vi "ProcessData.vi"() -> ()   [LabVIEW 2022 SP3]
panel:
  in  "Data Directory":path=path "C:/Users/LAV-UFSC-2023/Documents/LAV-TCC/Dados-Experimentos/Dados-Bancada-LABVIEW"
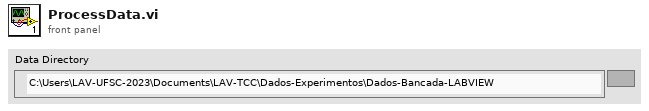
[diagram p1: front panel]
types:
  T1 = enum16{"open", "open or create", "create or replace", "create", "open (read-only)"}
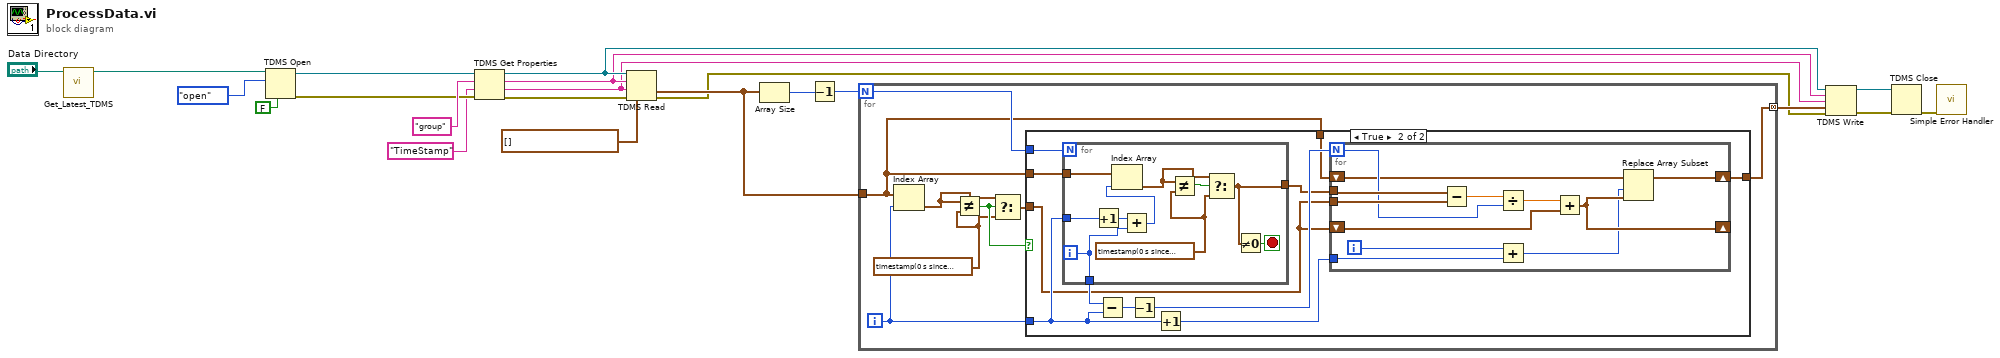
[diagram p0: block diagram]
diagram:
  n1 = call "Get_Latest_TDMS.vi"("Data Directory"="Data Directory") -> ("Latest_TDMS_File_Path"=w20:path)  [unwired: 10 in]
  n2 = TDMS Open(6:FALSE ("disable buffering? (T)"), 10:T1."open" ("operation (0:open)"), 11:w20) -> (0:w18:errorcluster, 3:w17:refnum<k34>)  [unwired: 4 in]
  n3 = TDMS Get Properties(8:w18, 9:"TimeStamp" ("group name (Untitled)"), 10:"group" ("group name (Untitled)"), 11:w17) -> (0:w13:errorcluster, 1:w5:string, 2:w7:string, 3:w8:refnum<k34>)  [unwired: 2 in, 2 out]
  n4 = TDMS Read(0:w8, 5:w7, 7:w5, 11:w13, 12:timestamp[] []) -> (10:w9:timestamp[], 15:w4:errorcluster)  [unwired: 3 in, 4 out]
  n5 = Array Size(array=w9) -> (size(s)=w11:i32)
  n6 = Decrement(x=w11) -> (x-1=w10:i32)
  n7 = for {
    N: w10 -> [w29]
    tunnel: w9 -> [w26]
    tunnel: [w25] -> w6 mode=concatenating
    i -> [w27]
    w22 = timestamp(0 s since 1904-01-01) ("f")
    n8 = Index Array(array=w26, index=w27) -> (element=w23:timestamp)
    n9 = Not Equal?(x=w23, y=w22) -> (x != y?=w24:bool)
    n10 = Select(t=w23, s=w24, f=w22) -> (s? t:f=w28:timestamp)
    n11 = case shown="True" w24 {
      tunnel: w29 -> [_ w41]
      tunnel: w26 -> [_ w40]
      tunnel: w28 -> [_ w34]
      tunnel: w27 -> [_ w35]
      tunnel: w26 -> [w30 w33]
      tunnel: [w30 w32] -> w25
      frame False {
      }
      frame True {
        n12 = for {
          N: w41 -> [_]
          tunnel: w40 -> [w63]
          tunnel: w35 -> [w54]
          tunnel: [w60] -> w31
          tunnel: [w59] -> w39
          i -> [w59]
          stop <- w61 stop-if-true
          w56 = timestamp(0 s since 1904-01-01) ("f")
          n13 = Increment(x=w54) -> (x+1=w55:i32)
          n14 = Add(x=w55, y=w59) -> (x+y=w62:i32)
          n15 = Index Array(array=w63, index=w62) -> (element=w57:timestamp)
          n16 = Not Equal?(x=w57, y=w56) -> (x != y?=w58:bool)
          n17 = Select(t=w57, s=w58, f=w56) -> (s? t:f=w60:timestamp)
          n18 = Not Equal To 0?(x=w60) -> (x != 0?=w61:bool)
        }
        n19 = Subtract(x=w39, y=w35) -> (x-y=w38:i32)
        n20 = Decrement(x=w38) -> (x-1=w37:i32)
        n21 = Increment(x=w35) -> (x+1=w36:i32)
        n22 = for {
          N: w37 -> [w50]
          tunnel: w31 -> [w53]
          tunnel: w34 -> [w52]
          shift-right: [w46] -> _
          shift-left: w34 -> [w49]
          tunnel: w36 -> [w48]
          shift-right: [w43] -> w32
          shift-left: w33 -> [w45]
          i -> [w47]
          n23 = Subtract(x=w53, y=w52) -> (x-y=w51:dbl)
          n24 = Divide(x=w51, y=w50) -> (x/y=w42:dbl)
          n25 = Add(x=w47, y=w48) -> (x+y=w44:i32)
          n26 = Add(x=w42, y=w49) -> (x+y=w46:timestamp)
          n27 = Replace Array Subset(array=w45, new element=w46, index=w44) -> (w43:timestamp[])
        }
      }
    }
  }
  n28 = TDMS Write(0:w8, 5:w7, 7:w5, 9:w6, 11:w4) -> (4:w2:refnum<k34>, 15:w3:errorcluster)  [unwired: 1 in, 2 out]
  n29 = TDMS Close(8:w3, 11:w2) -> (0:w1:errorcluster)  [unwired: 1 out]
  n30 = call <vilib>:"Simple Error Handler.vi"("error in (no error)"=w1) -> ()  [unwired: 4 in, 5 out]
